vi "触发环动报警入队列.vi"(9 "code":i32, 10 "告警详情":string, 11 "告警信息":string) -> ()   [LabVIEW 2016, in "环境动力监测库.lvlib"]
uses:
  Alarm interface/Alarm interface.lvlib
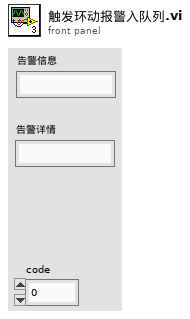
[diagram p1: front panel]
types:
  T1 = cluster{"componentParent":string, "equipVersion":string, string}
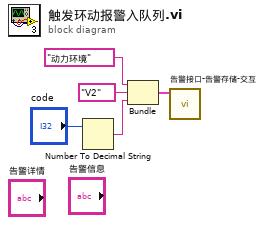
[diagram p0: block diagram]
diagram:
  n1 = Number To Decimal String(number="code") -> (decimal integer string=w2:string)  [unwired: 1 in]
  n2 = Bundle("componentParent"="动力环境", "equipVersion"="V2", w2) -> (w1:T1)  [unwired: 1 in]
  n3 = call "告警接口-告警存储-交互.vi"("筛选输入"=w1) -> ()  [unwired: 10 in, 1 out]
